vi "Calculate And Insert Biometry Average And Standard Deviation And State.vi"(8 "error in (no error)":errorcluster caption="错误输入（无错误）", 9 "L_Or_R":string, 10 "Measure_No":i64, 11 "connection reference":T1) -> (0 "error out":errorcluster caption="错误输出")   [LabVIEW 2015, in "Boimetry Processing.lvlib"]
doc: "计算多次生物参数测量结果的平均值、极值范围和测量结果错误判断。计算的结果添加到Biometry Average的Parameter、Standard Deviation和State数据库。\n输入：测量的第几次；左右眼选择。"
uses:
  Boimetry Processing.lvlib
  <vilib>/addons/database/Connection.llb/Conn ObjectReference.ctl
  Database Processing/Support/Table/Biometry Average Standard Deviation.ctl
  Database Processing/Support/Table/Biometry Average Parameter.ctl
  Database Processing/Support/Table/Biometry Average Attribute.ctl
  Database Processing/Support/Table/Biometry Average State.ctl
  <vilib>/Analysis/baseanly.llb/Mean (DBL).vi
  Database Processing/Database Processing.lvlib
  <vilib>/addons/database/NI_Database_API.lvlib
  <vilib>/Analysis/NI_AALBase.lvlib
panel:
  # "Busy"
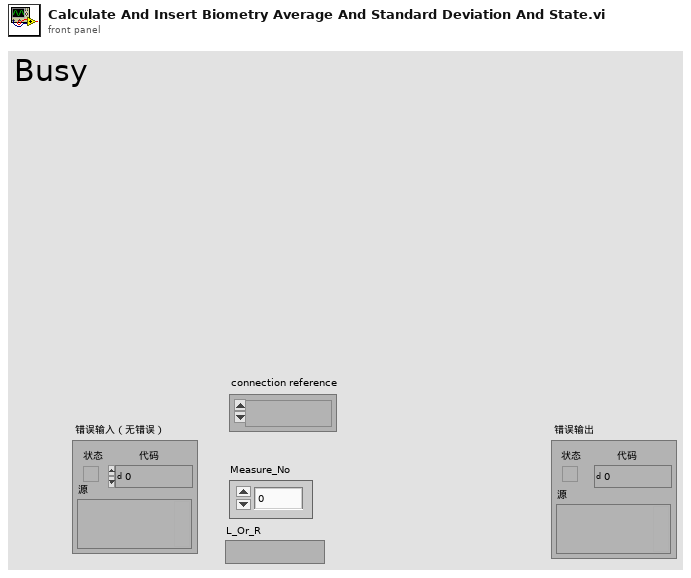
[diagram p1: front panel]
types:
  T1 = typedef "NI_Database_API.lvlib/Conn ObjectReference.ctl" = refnum<k1>
  T2 = typedef "Database Processing.lvlib/Biometry Average State.ctl" = cluster{"Parameter_ID":i64, "Central_Corneal_Thickness_State":string, "Anterior_Chamber_Depth_State":string, "Len_Thickness_State":string, "Retinal_Thickness_State":string, "Axis_Length_State":string, "Pupil_Diameter_State":string, "White_To_White_State":string, "Keratometric_flat_State":string, "Keratometric_steep_State":string}
  T3 = typedef "Database Processing.lvlib/Biometry Average Attribute.ctl" = cluster{"Parameter_ID":i64, "Measure_No":i64, "L_Or_R":string}
  T4 = typedef "Database Processing.lvlib/Biometry Average Parameter.ctl" = cluster{"Parameter_ID":i64, "Central_Corneal_Thickness":sgl, "Anterior_Chamber_Depth":sgl, "Len_Thickness":sgl, "Retinal_Thickness":sgl, "Axis_Length":sgl, "Pupil_Diameter":sgl, "PCX":sgl, "PCY":sgl, "White_To_White":sgl, "ICX":sgl, "ICY":sgl, "Keratometric_flat":sgl, "Keratometric_steep":sgl, "Keratometric_Axis(flat)":sgl, "Keratometric_Axis(steep)":sgl, "Keratometric_AST":sgl}
  T5 = typedef "Database Processing.lvlib/Biometry Average Standard Deviation.ctl" = cluster{"Parameter_ID":i64, "Central_Corneal_Thickness":sgl, "Anterior_Chamber_Depth":sgl, "Len_Thickness":sgl, "Retinal_Thickness":sgl, "Axis_Length":sgl, "Pupil_Diameter":sgl, "PCX":sgl, "PCY":sgl, "White_To_White":sgl, "ICX":sgl, "ICY":sgl, "Keratometric_flat":sgl, "Keratometric_steep":sgl, "Keratometric_Axis(flat)":sgl, "Keratometric_Axis(steep)":sgl, "Keratometric_AST":sgl}
  T6 = typedef "Database Processing.lvlib/Biometry Attribute.ctl" = cluster{"Measure_ID":i64, "Measure_No":i64, "Ordinal":i64, "L_Or_R":string}
  T7 = typedef "Database Processing.lvlib/Biometry Parameter.ctl" = cluster{"Measure_ID":i64, "Central_Corneal_Thickness":sgl, "Anterior_Chamber_Depth":sgl, "Len_Thickness":sgl, "Retinal_Thickness":sgl, "Axis_Length":sgl, "Pupil_Diameter":sgl, "PCX":sgl, "PCY":sgl, "White_To_White":sgl, "ICX":sgl, "ICY":sgl, "Keratometric_flat":sgl, "Keratometric_steep":sgl, "Keratometric_Axis(flat)":sgl, "Keratometric_Axis(steep)":sgl, "Keratometric_AST":sgl}
  T8 = typedef "Database Processing.lvlib/Biometry State.ctl" = cluster{"Measure_ID":i64, "Central_Corneal_Thickness_State":string, "Anterior_Chamber_Depth_State":string, "Len_Thickness_State":string, "Retinal_Thickness_State":string, "Axis_Length_State":string, "Pupil_Diameter_State":string, "White_To_White_State":string, "Keratometric_flat_State":string, "Keratometric_steep_State":string}
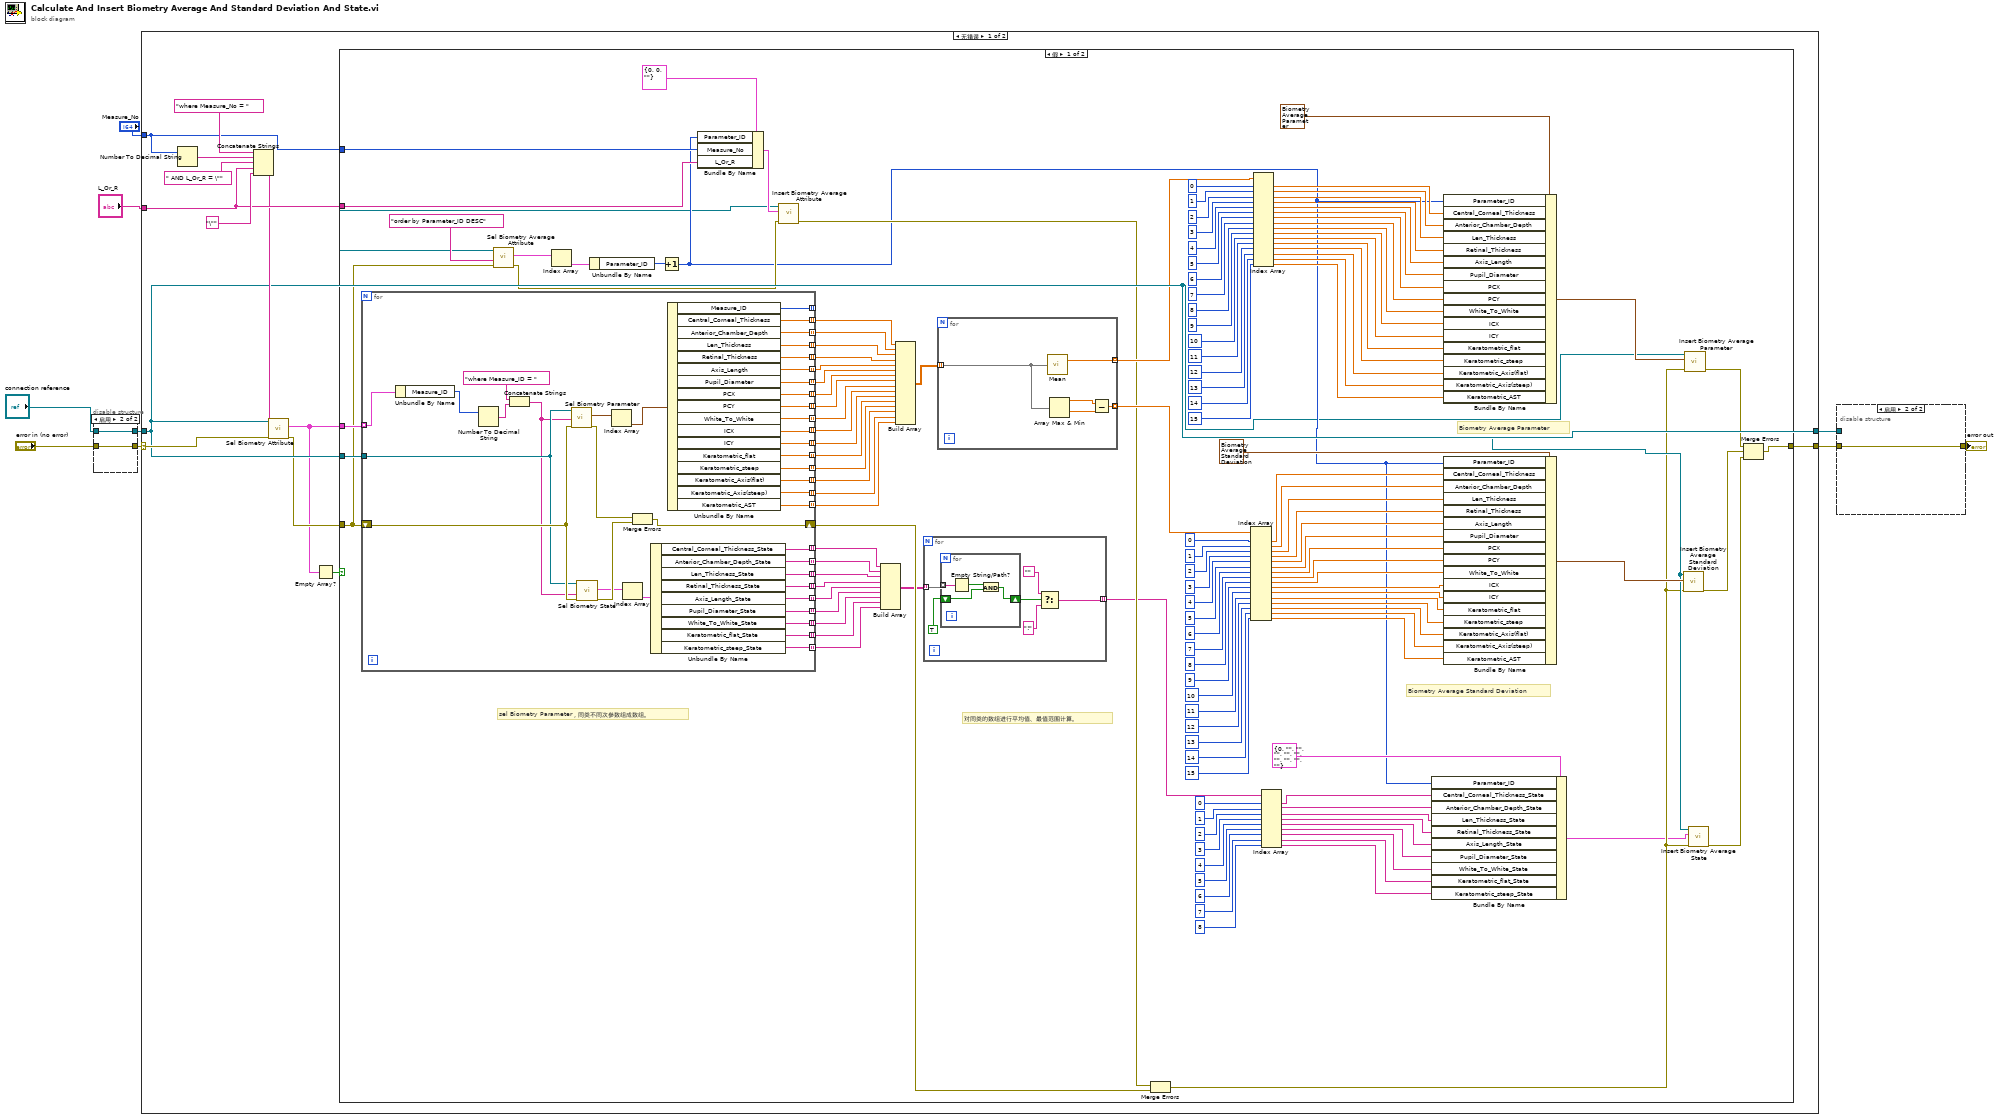
[diagram p0: block diagram]
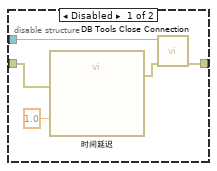
[diagram p2: hidden frame]
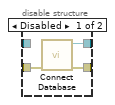
[diagram p3: hidden frame]
diagram:
  n1 = disable-structure shown="启用" {
    disable-tunnel: [w12 w14] -> w9
    disable-tunnel: "error in (no error)" -> [w11 w13]
    disable-tunnel: [w10 w13] -> w7
    disable-tunnel: "connection reference" -> [_ w14]
    frame Disabled {
      n2 = call "Connect Database.vi"("error in (no error)"=w11) -> ("error out"=w10:errorcluster, "connection reference"=w12:T1)  [unwired: 9 in]
    }
    frame Enabled {
    }
  }
  n3 = case shown="无错误" w7 {
    selector: w7 -> [w23 w223]
    tunnel: [w20 w223] -> w5
    tunnel: "Measure_No" -> [w22 _]
    tunnel: w9 -> [w18 w222]
    tunnel: [w18 w222] -> w4
    tunnel: "L_Or_R" -> [w21 _]
    frame No Error {
      n4 = Number To Decimal String(number=w22) -> (decimal integer string=w24:string)  [unwired: 1 in]
      n5 = Concatenate Strings("where Measure_No = " ("数据库配置.Condition"), w24, " AND L_Or_R = \"" ("字符串"), w21, "\"" ("字符串")) -> (w19:string)
      n6 = call "Sel Biometry Attribute.vi"("error in (no error)"=w23, "condition"=w19, "connection reference"=w18) -> ("error out"=w17:errorcluster, "Biometry Attribute"=w15:T6[])  [unwired: 7 in]
      n7 = Empty Array?(array=w15) -> (empty?=w16:bool)
      n8 = case shown="假" w16 {
        tunnel: w15 -> [w165 _]
        tunnel: w22 -> [w73 _]
        tunnel: w21 -> [w72 _]
        tunnel: [w64 w221] -> w20
        tunnel: w18 -> [w32 _]
        tunnel: w17 -> [w28 w221]
        frame False {
          # "Biometry Average Parameter"
          # "Biometry Average Standard Deviation"
          # "对同类的数组进行平均值、最值范围计算。"
          # "sel Biometry Parameter，同类不同次参数组成数组。"
          n9 = for {
            tunnel: w165 -> [w217] mode=indexing
            shift-right: [w181] -> w68
            shift-left: w28 -> [w188]
            tunnel: w32 -> [w183]
            tunnel: [w214] -> w164 mode=indexing
            tunnel: [w213] -> w163 mode=indexing
            tunnel: [w212] -> w162 mode=indexing
            tunnel: [w211] -> w161 mode=indexing
            tunnel: [w210] -> w160 mode=indexing
            tunnel: [w209] -> w159 mode=indexing
            tunnel: [w208] -> w158 mode=indexing
            tunnel: [w207] -> w157 mode=indexing
            tunnel: [w206] -> w156 mode=indexing
            tunnel: [w205] -> _ mode=indexing
            tunnel: [w204] -> w152 mode=indexing
            tunnel: [w203] -> w151 mode=indexing
            tunnel: [w202] -> w150 mode=indexing
            tunnel: [w201] -> w149 mode=indexing
            tunnel: [w200] -> w148 mode=indexing
            tunnel: [w199] -> w147 mode=indexing
            tunnel: [w198] -> w146 mode=indexing
            tunnel: [w197] -> w63 mode=indexing
            tunnel: [w196] -> w62 mode=indexing
            tunnel: [w195] -> w61 mode=indexing
            tunnel: [w194] -> w60 mode=indexing
            tunnel: [w193] -> w59 mode=indexing
            tunnel: [w192] -> w58 mode=indexing
            tunnel: [w191] -> w57 mode=indexing
            tunnel: [w190] -> w56 mode=indexing
            tunnel: [w189] -> w55 mode=indexing
            n10 = Unbundle By Name(w217) -> ("Measure_ID"=w218:i64)
            n11 = Number To Decimal String(number=w218) -> (decimal integer string=w220:string)  [unwired: 1 in]
            n12 = Concatenate Strings("where Measure_ID = " ("数据库配置.Condition"), w220) -> (w182:string)
            n13 = call "Sel Biometry Parameter.vi"("error in (no error)"=w188, "condition"=w182, "connection reference"=w183) -> ("error out"=w187:errorcluster, "Biometry Parameter"=w216:T7[])  [unwired: 7 in]
            n14 = call "Sel Biometry State.vi"("error in (no error)"=w188, "condition"=w182, "connection reference"=w183) -> ("error out"=w186:errorcluster, "Biometry State"=w185:T8[])  [unwired: 7 in]
            n15 = Index Array(array=w216) -> (element=w215:T7)  [unwired: 1 in]
            n16 = Index Array(array=w185) -> (element=w184:T8)  [unwired: 1 in]
            n17 = Merge Errors(w187, w186) -> (w181:errorcluster)
            n18 = Unbundle By Name(w184) -> ("Central_Corneal_Thickness_State"=w197:string, "Anterior_Chamber_Depth_State"=w196:string, "Len_Thickness_State"=w195:string, "Retinal_Thickness_State"=w194:string, "Axis_Length_State"=w193:string, "Pupil_Diameter_State"=w192:string, "White_To_White_State"=w191:string, "Keratometric_flat_State"=w190:string, "Keratometric_steep_State"=w189:string)
            n19 = Unbundle By Name(w215) -> ("Measure_ID"=w205:i64, "Central_Corneal_Thickness"=w214:sgl, "Anterior_Chamber_Depth"=w213:sgl, "Len_Thickness"=w212:sgl, "Retinal_Thickness"=w211:sgl, "Axis_Length"=w210:sgl, "Pupil_Diameter"=w209:sgl, "PCX"=w208:sgl, "PCY"=w207:sgl, "White_To_White"=w206:sgl, "ICX"=w204:sgl, "ICY"=w203:sgl, "Keratometric_flat"=w202:sgl, "Keratometric_steep"=w201:sgl, "Keratometric_Axis(flat)"=w200:sgl, "Keratometric_Axis(steep)"=w199:sgl, "Keratometric_AST"=w198:sgl)
          }
          n20 = call "Sel Biometry Average Attribute.vi"("error in (no error)"=w28, "condition"="order by Parameter_ID DESC", "connection reference"=w32) -> ("error out"=w70:errorcluster, "Biometry Average Attribute"=w76:T3[])  [unwired: 7 in]
          n21 = Index Array(array=w76) -> (element=w75:T3)  [unwired: 1 in]
          n22 = Unbundle By Name(w75) -> ("Parameter_ID"=w69:i64)
          n23 = Increment(x=w69) -> (x+1=w42:i64)
          n24 = Bundle By Name(cluster=T3 {"Parameter_ID"=0, "Measure_No"=0, "L_Or_R"=""} ("Biometry Average Attribute"), "Parameter_ID"=w42, "Measure_No"=w73, "L_Or_R"=w72) -> (w71:T3)
          n25 = call "Insert Biometry Average Attribute.vi"("error in (no error)"=w70, "Biometry Average Attribute Input"=w71, "connection reference"=w32) -> ("error out"=w67:errorcluster)  [unwired: 8 in]
          n26 = Build Array(w63, w62, w61, w60, w59, w58, w57, w56, w55) -> (w54:string[][])
          n27 = Build Array(w164, w163, w162, w161, w160, w159, w158, w157, w156, w152, w151, w150, w149, w148, w147, w146) -> (w155:sgl[][])
          n28 = for {
            tunnel: w54 -> [w171] mode=indexing
            tunnel: [w170] -> w44 mode=indexing
            n29 = for {
              tunnel: w171 -> [w175] mode=indexing
              shift-right: [w173] -> w168
              shift-left: TRUE -> [w172]
              n30 = Empty String/Path?(string/path=w175) -> (empty?=w174:bool)
              n31 = And(x=w174, y=w172) -> (x .and. y?=w173:bool)
            }
            n32 = Select(t="", s=w168, f="!") -> (s? t:f=w170:string)
          }
          n33 = for {
            tunnel: w155 -> [w180] mode=indexing
            tunnel: [w179] -> w113 mode=indexing
            tunnel: [w178] -> w112 mode=indexing
            n34 = call-poly <vilib>:"Mean.vi"("X"=w180) -> ("mean"=w179:dbl)  [unwired: 1 out]
            n35 = Array Max & Min(array=w180) -> (max value=w177:sgl, min value=w176:sgl)  [unwired: 2 out]
            n36 = Subtract(x=w177, y=w176) -> (x-y=w178:sgl)
          }
          n37 = Merge Errors(w67, w68) -> (w31:errorcluster)
          n38 = Index Array(array=w112, index #1=0 ("索引"), index #2=1 ("索引"), index #3=2 ("索引"), index #4=3 ("索引"), index #5=4 ("索引"), index #6=5 ("索引"), index #7=6 ("索引"), index #8=7 ("索引"), index #9=8 ("索引"), index #10=9 ("索引"), index #11=10 ("索引"), index #12=11 ("索引"), index #13=12 ("索引"), index #14=13 ("索引"), index #15=14 ("索引"), index #16=15 ("索引")) -> (element #1=w95:sgl, element #2=w94:sgl, element #3=w93:sgl, element #4=w92:sgl, element #5=w91:sgl, element #6=w90:sgl, element #7=w89:sgl, element #8=w88:sgl, element #9=w87:sgl, element #10=w86:sgl, element #11=w85:sgl, element #12=w84:sgl, element #13=w83:sgl, element #14=w82:sgl, element #15=w81:sgl, element #16=w80:sgl)
          n39 = Index Array(array=w113, index #1=0 ("索引"), index #2=1 ("索引"), index #3=2 ("索引"), index #4=3 ("索引"), index #5=4 ("索引"), index #6=5 ("索引"), index #7=6 ("索引"), index #8=7 ("索引"), index #9=8 ("索引"), index #10=9 ("索引"), index #11=10 ("索引"), index #12=11 ("索引"), index #13=12 ("索引"), index #14=13 ("索引"), index #15=14 ("索引"), index #16=15 ("索引")) -> (element #1=w111:dbl, element #2=w110:dbl, element #3=w109:dbl, element #4=w108:dbl, element #5=w107:dbl, element #6=w106:dbl, element #7=w105:dbl, element #8=w104:dbl, element #9=w103:dbl, element #10=w102:dbl, element #11=w101:dbl, element #12=w100:dbl, element #13=w99:dbl, element #14=w98:dbl, element #15=w97:dbl, element #16=w96:dbl)
          n40 = Index Array(array=w44, index #1=0 ("索引"), index #2=1 ("索引"), index #3=2 ("索引"), index #4=3 ("索引"), index #5=4 ("索引"), index #6=5 ("索引"), index #7=6 ("索引"), index #8=7 ("索引"), index #9=8 ("索引")) -> (element #1=w41:string, element #2=w40:string, element #3=w39:string, element #4=w38:string, element #5=w37:string, element #6=w36:string, element #7=w35:string, element #8=w34:string, element #9=w33:string)
          n41 = Bundle By Name(cluster=T2 {"Parameter_ID"=0, "Central_Corneal_Thickness_State"="", "Anterior_Chamber_Depth_State"="", "Len_Thickness_State"="", "Retinal_Thickness_State"="", "Axis_Length_State"="", "Pupil_Diameter_State"="", "White_To_White_State"="", "Keratometric_flat_State"="", "Keratometric_steep_State"=""} ("Biometry Average State"), "Parameter_ID"=w42, "Central_Corneal_Thickness_State"=w41, "Anterior_Chamber_Depth_State"=w40, "Len_Thickness_State"=w39, "Retinal_Thickness_State"=w38, "Axis_Length_State"=w37, "Pupil_Diameter_State"=w36, "White_To_White_State"=w35, "Keratometric_flat_State"=w34, "Keratometric_steep_State"=w33) -> (w30:T2)
          n42 = Bundle By Name(cluster=T4 {"Parameter_ID"=0, "Central_Corneal_Thickness"=0.0, "Anterior_Chamber_Depth"=0.0, "Len_Thickness"=0.0, "Retinal_Thickness"=0.0, "Axis_Length"=0.0, "Pupil_Diameter"=0.0, "PCX"=0.0, "PCY"=0.0, "White_To_White"=0.0, "ICX"=0.0, "ICY"=0.0, "Keratometric_flat"=0.0, "Keratometric_steep"=0.0, "Keratometric_Axis(flat)"=0.0, "Keratometric_Axis(steep)"=0.0, "Keratometric_AST"=0.0} ("Biometry_Average"), "Parameter_ID"=w42, "Central_Corneal_Thickness"=w111, "Anterior_Chamber_Depth"=w110, "Len_Thickness"=w109, "Retinal_Thickness"=w108, "Axis_Length"=w107, "Pupil_Diameter"=w106, "PCX"=w105, "PCY"=w104, "White_To_White"=w103, "ICX"=w102, "ICY"=w101, "Keratometric_flat"=w100, "Keratometric_steep"=w99, "Keratometric_Axis(flat)"=w98, "Keratometric_Axis(steep)"=w97, "Keratometric_AST"=w96) -> (w79:T4)
          n43 = Bundle By Name(cluster=T5 {"Parameter_ID"=0, "Central_Corneal_Thickness"=0.0, "Anterior_Chamber_Depth"=0.0, "Len_Thickness"=0.0, "Retinal_Thickness"=0.0, "Axis_Length"=0.0, "Pupil_Diameter"=0.0, "PCX"=0.0, "PCY"=0.0, "White_To_White"=0.0, "ICX"=0.0, "ICY"=0.0, "Keratometric_flat"=0.0, "Keratometric_steep"=0.0, "Keratometric_Axis(flat)"=0.0, "Keratometric_Axis(steep)"=0.0, "Keratometric_AST"=0.0} ("Biometry Average Standard Deviation"), "Parameter_ID"=w42, "Central_Corneal_Thickness"=w95, "Anterior_Chamber_Depth"=w94, "Len_Thickness"=w93, "Retinal_Thickness"=w92, "Axis_Length"=w91, "Pupil_Diameter"=w90, "PCX"=w89, "PCY"=w88, "White_To_White"=w87, "ICX"=w86, "ICY"=w85, "Keratometric_flat"=w84, "Keratometric_steep"=w83, "Keratometric_Axis(flat)"=w82, "Keratometric_Axis(steep)"=w81, "Keratometric_AST"=w80) -> (w78:T5)
          n44 = call "Insert Biometry Average Standard Deviation.vi"("error in (no error)"=w31, "Biometry Average Standard Deviation"=w78, "connection reference"=w32) -> ("error out"=w65:errorcluster)  [unwired: 8 in]
          n45 = call "Insert Biometry Average Parameter.vi"("error in (no error)"=w31, "Biometry_Average Inpute"=w79, "connection reference"=w32) -> ("error out"=w66:errorcluster)  [unwired: 8 in]
          n46 = call "Insert Biometry Average State.vi"("error in (no error)"=w31, "Biometry Average State"=w30, "connection reference"=w32) -> ("error out"=w29:errorcluster)  [unwired: 8 in]
          n47 = Merge Errors(w66, w65, w29) -> (w64:errorcluster)
        }
        frame True {
        }
      }
    }
    frame Error {
    }
  }
  n48 = disable-structure shown="启用" {
    disable-tunnel: w5 -> [w225 w229]
    disable-tunnel: [w228 w229] -> w3
    disable-tunnel: w4 -> [w227 _]
    frame Disabled {
      n49 = call "时间延迟"("error in (no error)"=w225, "Delay Time (s)"=1.0) -> ("error out"=w224:errorcluster)  [unwired: 9 in]
      n50 = call <vilib>:"DB Tools Close Connection.vi"("error in (no error)"=w224, "connection reference"=w227) -> ("error out"=w228:errorcluster)  [unwired: 5 in]
    }
    frame Enabled {
    }
  }
  "error out" <- w3
